vi "WriteData.vi"(8 "error in":errorcluster, 11 "refnum in":refnum<file>) -> (0 "error out":errorcluster, 3 "refnum out":refnum<file>)   [LabVIEW 2017]
doc: "Logs data to csv file on roborio"
uses:
  <vilib>/Rock Robotics/Network Tables/NT Read Number.vi
  <vilib>/Rock Robotics/Network Tables/NT Read Boolean.vi
  <vilib>/Rock Robotics/Network Tables/NT Read String.vi
  Robot Global Data.vi
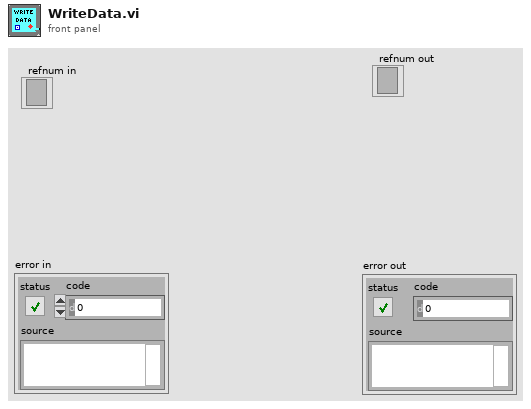
[diagram p1: front panel]
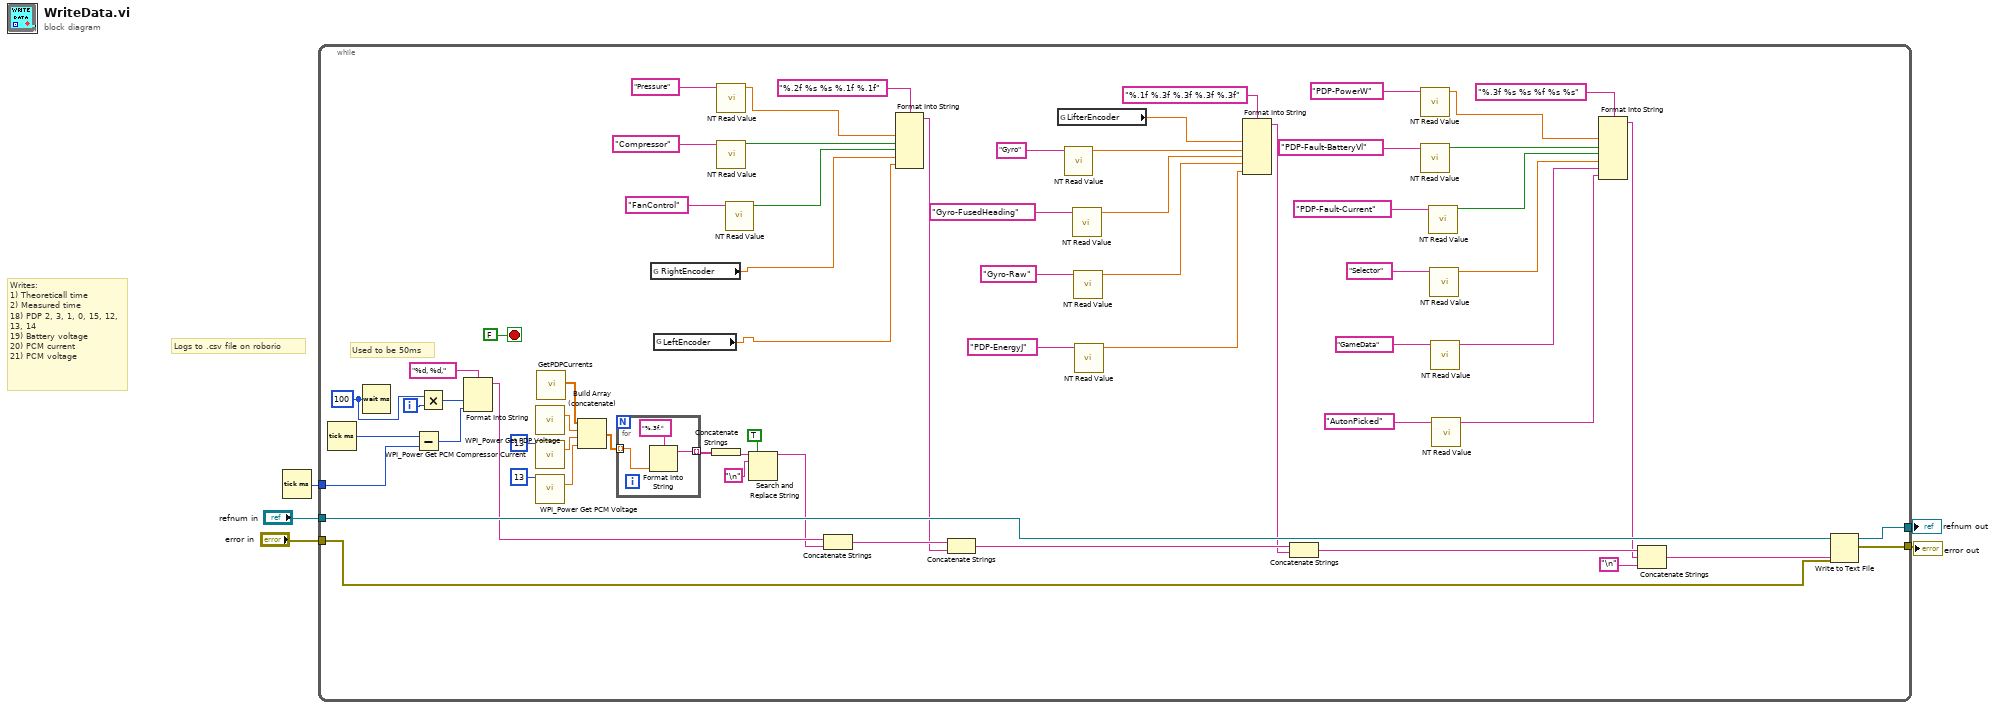
[diagram p0: block diagram]
diagram:
  # "Logs to .csv file on roborio"
  # "Writes:\n1) Theoreticall time\n2) Measured time\n18) PDP 2, 3, 1, 0, 15, 12,\n13, 14\n19) Battery voltage\n20) PCM current\n21) PCM voltage"
  n1 = Tick Count (ms)() -> (millisecond timer value=w1:u32)
  n2 = while {
    tunnel: "error in" -> [w68]
    tunnel: "refnum in" -> [w67]
    tunnel: [w65] -> w3
    tunnel: [w66] -> w2
    tunnel: w1 -> [w64]
    i -> [w69]
    stop <- FALSE stop-if-true
    w63 = u32 100 ("milliseconds to wait")
    # "Used to be 50ms"
    n3 = Tick Count (ms)() -> (millisecond timer value=w51:u32)
    n4 = Wait (ms)(milliseconds to wait=w63) -> ()  [unwired: 1 out]
    n5 = Subtract(x=w51, y=w64) -> (x-y=w50:u32)
    n6 = Multiply(x=w63, y=w69) -> (x*y=w62:u32)
    n7 = Format Into String(format string="%d, %d,", w62, w50) -> (resulting string=w48:string)  [unwired: 2 in, 1 out]
    n8 = call <vilib>:"WPI_Power Get PDP Voltage.vi"() -> ("voltage (V)"=w58:dbl)  [unwired: 14 in, 1 out]
    n9 = call <vilib>:"WPI_Power Get PCM Compressor Current.vi"("Pneumatics Control Module (0)"=u8 13) -> ("current (A)"=w54:dbl)  [unwired: 13 in, 1 out]
    n10 = call <vilib>:"WPI_Power Get PCM Voltage.vi"("Pneumatics Control Module (0)"=u8 13) -> ("Input Voltage"=w53:dbl)  [unwired: 12 in, 2 out]
    n11 = call "GetPDPCurrents.vi"() -> ("PDP Currents"=w52:dbl[])  [unwired: 11 in]
    n12 = Build Array (concatenate)(w52, w58, w54, w53) -> (w57:dbl[])
    n13 = for {
      tunnel: w57 -> [w73] mode=indexing
      tunnel: [w71] -> w56 mode=indexing
      n14 = Format Into String(format string="%.3f,", w73) -> (resulting string=w71:string)  [unwired: 2 in, 1 out]
    }
    n15 = global read "Robot Global Data.vi" "RightEncoder"() -> (w10:dbl)
    n16 = global read "Robot Global Data.vi" "LeftEncoder"() -> (w11:dbl)
    n17 = Concatenate Strings(w56) -> (w55:string)
    n18 = call-poly <vilib>:"NT Read Value.vi"("Name"="Pressure") -> ("Numeric"=w42:dbl)  [unwired: 9 in, 1 out]
    n19 = call-poly <vilib>:"NT Read Value.vi"("Name"="Compressor") -> ("Boolean"=w38:bool)  [unwired: 9 in, 1 out]
    n20 = call-poly <vilib>:"NT Read Value.vi"("Name"="FanControl") -> ("Boolean"=w37:bool)  [unwired: 9 in, 1 out]
    n21 = Search and Replace String(replace all?=TRUE ("replace all? (F)"), input string=w55, search string="\n") -> (result string=w47:string)  [unwired: 5 in, 3 out]
    n22 = Concatenate Strings(w48, w47) -> (w49:string)
    n23 = Format Into String(format string="%.2f %s %s %.1f %.1f", w42, w38, w37, w10, w11) -> (resulting string=w43:string)  [unwired: 2 in, 1 out]
    n24 = Concatenate Strings(w49, w43) -> (w44:string)
    n25 = global read "Robot Global Data.vi" "LifterEncoder"() -> (w12:dbl)
    n26 = call-poly <vilib>:"NT Read Value.vi"("Name"="Gyro") -> ("Numeric"=w33:dbl)  [unwired: 9 in, 1 out]
    n27 = call-poly <vilib>:"NT Read Value.vi"("Name"="Gyro-FusedHeading") -> ("Numeric"=w32:dbl)  [unwired: 9 in, 1 out]
    n28 = call-poly <vilib>:"NT Read Value.vi"("Name"="Gyro-Raw") -> ("Numeric"=w31:dbl)  [unwired: 9 in, 1 out]
    n29 = call-poly <vilib>:"NT Read Value.vi"("Name"="PDP-EnergyJ") -> ("Numeric"=w30:dbl)  [unwired: 9 in, 1 out]
    n30 = Format Into String(format string="%.1f %.3f %.3f %.3f %.3f", w12, w33, w32, w31, w30) -> (resulting string=w27:string)  [unwired: 2 in, 1 out]
    n31 = Concatenate Strings(w44, w27) -> (w28:string)
    n32 = call-poly <vilib>:"NT Read Value.vi"("Name"="PDP-PowerW") -> ("Numeric"=w22:dbl)  [unwired: 9 in, 1 out]
    n33 = call-poly <vilib>:"NT Read Value.vi"("Name"="PDP-Fault-BatteryVl") -> ("Boolean"=w23:bool)  [unwired: 9 in, 1 out]
    n34 = call-poly <vilib>:"NT Read Value.vi"("Name"="PDP-Fault-Current") -> ("Boolean"=w24:bool)  [unwired: 9 in, 1 out]
    n35 = call-poly <vilib>:"NT Read Value.vi"("Name"="Selector") -> ("Numeric"=w25:dbl)  [unwired: 9 in, 1 out]
    n36 = call-poly <vilib>:"NT Read Value.vi"("Name"="GameData") -> ("String"=w26:string)  [unwired: 9 in, 1 out]
    n37 = call-poly <vilib>:"NT Read Value.vi"("Name"="AutonPicked") -> ("String"=w13:string)  [unwired: 9 in, 1 out]
    n38 = Format Into String(format string="%.3f %s %s %f %s %s", w22, w23, w24, w25, w26, w13) -> (resulting string=w15:string)  [unwired: 2 in, 1 out]
    n39 = Concatenate Strings(w28, w15, "\n") -> (w16:string)
    n40 = Write to Text File(file (use dialog)=w67, text=w16, error in=w68) -> (refnum out=w65:refnum<file>, error out=w66:errorcluster)  [unwired: 1 in, 1 out]
  }
  "refnum out" <- w3
  "error out" <- w2
